vi "MCP2221_Close.vi"(8 "error in":errorcluster, 9 "handle in":i32) -> (0 "error out":errorcluster, 1 "handle out":i32, 3 "return type":i32)   [LabVIEW 2025]
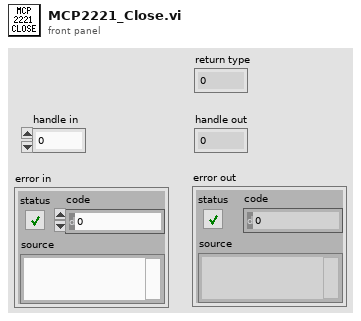
[diagram p1: front panel]
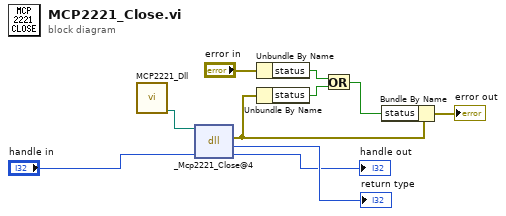
[diagram p0: block diagram]
diagram:
  n1 = call "MCP2221_Dll.vi"() -> ("dll path"=w7:path)  [unwired: 11 in]
  n2 = dll-call lib="?" fn="_Mcp2221_Close@4"(path in=w7, "handle"="handle in") -> (error out=w4:errorcluster, "return type"=→"return type":i32, "handle"=→"handle out":i32)  [unwired: 2 in, 1 out]
  n3 = Unbundle By Name("error in") -> ("status"=w3:bool)
  n4 = Unbundle By Name(w4) -> ("status"=w2:bool)
  n5 = Or(x=w3, y=w2) -> (x .or. y?=w1:bool)
  n6 = Bundle By Name(cluster=w4, "status"=w1) -> (→"error out":errorcluster)
